vi "灰度图像平滑去毛刺处理.vi"(9 "滤波方法选择":enum16{"中值滤波", "平滑滤波"}(ring), 11 "Image":T1) -> (3 "Image Out":T1)   [LabVIEW 2018]
uses:
  <vilib>/vision/Image Controls.llb/IMAQ Image.ctl
  <vilib>/vision/NI_Vision_Development_Module.lvlib
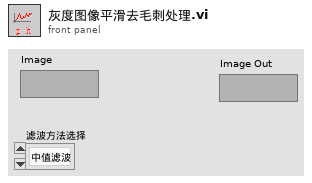
[diagram p1: front panel]
types:
  T1 = typedef "IMAQ Image.ctl" = refnum<image>
  T2 = cluster{bool, bool, bool, bool, bool, bool, bool, bool}
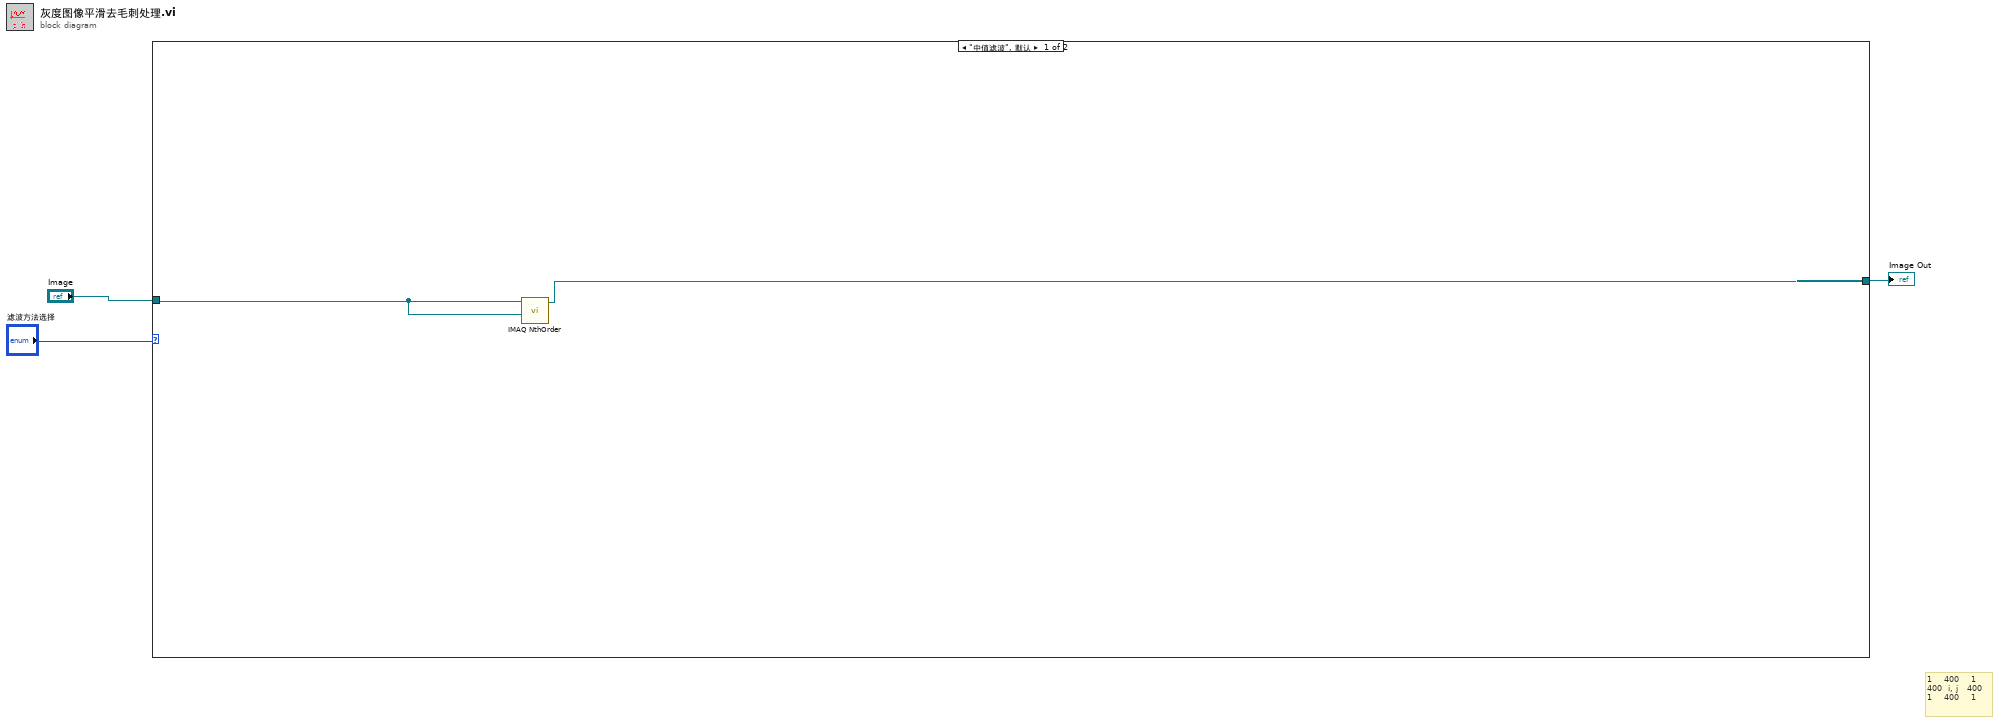
[diagram p0: block diagram]
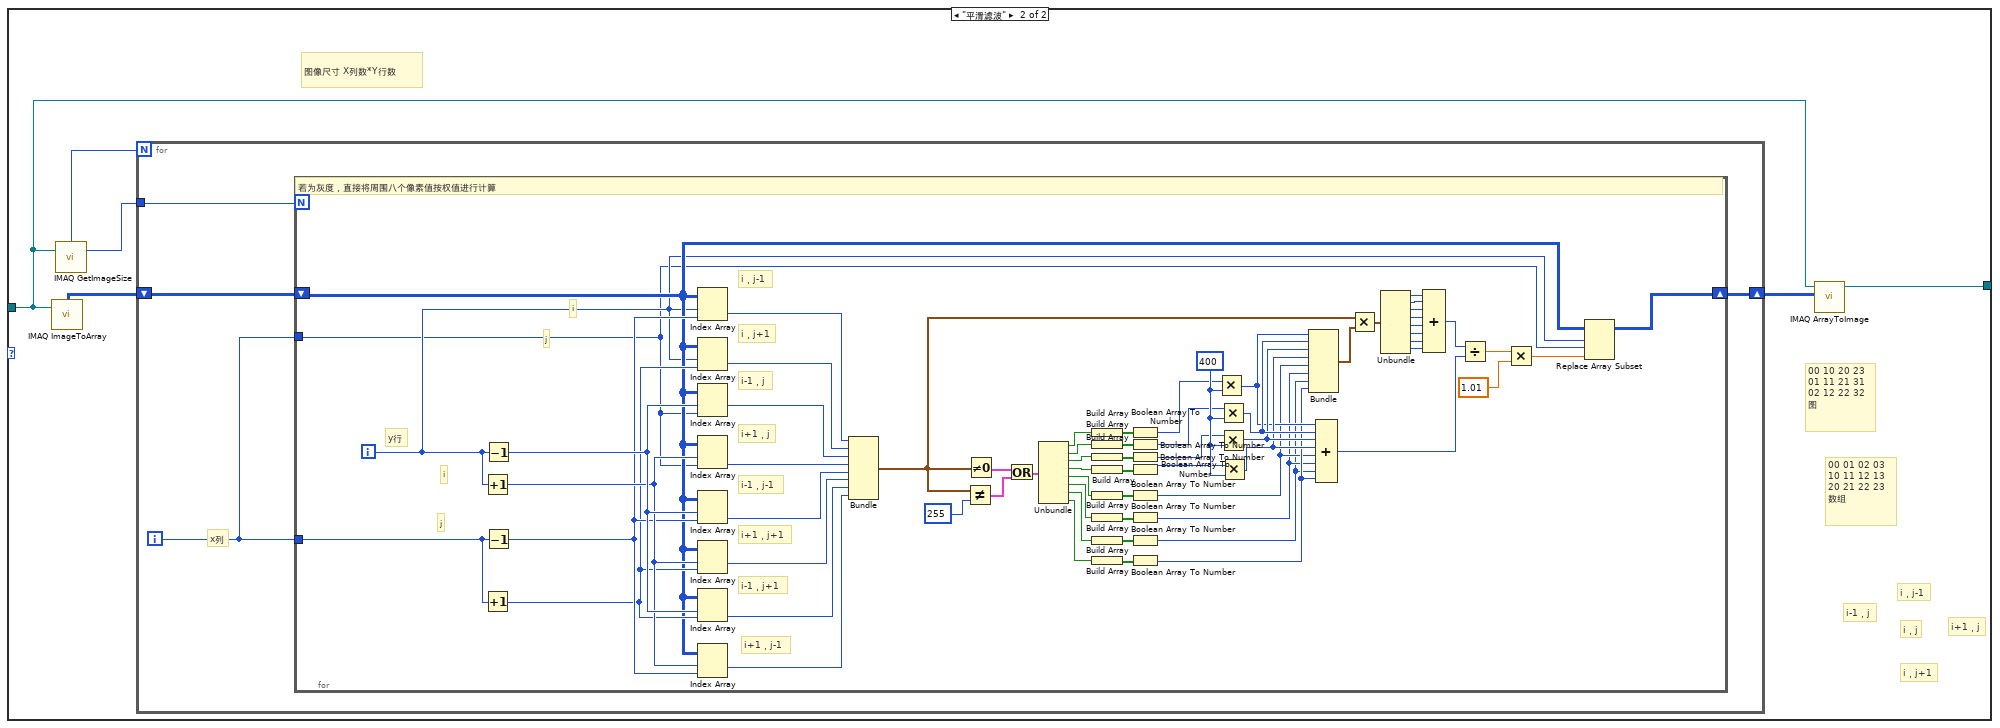
[diagram p2: hidden frame]
diagram:
  # "1    400    1\n400  i, j   400\n1    400    1"
  n1 = case shown="\"中值滤波\", 默认" "滤波方法选择" {
    tunnel: [w4 w11] -> w3
    tunnel: "Image" -> [w5 w8]
    frame "中值滤波", Default {
      n2 = call "IMAQ NthOrder"("Image Src"=w5, "Image Dst"=w5) -> ("Image Dst Out"=w4:T1)  [unwired: 5 in, 1 out]
    }
    frame "平滑滤波" {
      # "i+1，j"
      # "i，j+1"
      # "i，j"
      # "i，j-1"
      # "00 10 20 23\n01 11 21 31\n02 12 22 32\n图"
      # "i-1，j"
      # "00 01 02 03\n10 11 12 13\n20 21 22 23\n数组"
      # "图像尺寸 X列数*Y行数"
      n3 = call "IMAQ ImageToArray"("Image"=w8) -> ("Image Pixels (U8)"=w9:u8[][])  [unwired: 3 in, 4 out]
      n4 = call "IMAQ GetImageSize"("Image"=w8) -> ("Y Resolution"=w7:i32, "X Resolution"=w6:i32)  [unwired: 3 in, 1 out]
      n5 = for {
        N: w6 -> [_]
        shift-right: [w14] -> w10
        shift-left: w9 -> [w15]
        tunnel: w7 -> [w13]
        i -> [w12]
        # "x列"
        n6 = for {
          N: w13 -> [_]
          shift-right: [w79] -> w14
          shift-left: w15 -> [w45]
          tunnel: w12 -> [w78]
          tunnel: w12 -> [w43]
          i -> [w44]
          w75 = u32 400 ("y")
          # "i+1，j-1"
          # "i-1，j+1"
          # "i+1，j+1"
          # "i-1，j-1"
          # "i-1，j"
          # "i+1，j"
          # "i，j+1"
          # "i，j-1"
          # "j"
          # "i"
          # "i"
          # "j"
          # "y行"
          # "若为灰度，直接将周围八个像素值按权值进行计算"
          n7 = Increment(x=w44) -> (x+1=w80:i32)
          n8 = Increment(x=w78) -> (x+1=w76:i32)
          n9 = Decrement(x=w44) -> (x-1=w81:i32)
          n10 = Decrement(x=w78) -> (x-1=w77:i32)
          n11 = Index Array(array=w45, index (row)=w44, index (col)=w77) -> (element=w53:u8)
          n12 = Index Array(array=w45, index (row)=w44, index (col)=w76) -> (element=w52:u8)
          n13 = Index Array(array=w45, index (row)=w81, index (col)=w43) -> (element=w51:u8)
          n14 = Index Array(array=w45, index (row)=w80, index (col)=w43) -> (element=w50:u8)
          n15 = Index Array(array=w45, index (row)=w81, index (col)=w77) -> (element=w49:u8)
          n16 = Index Array(array=w45, index (row)=w80, index (col)=w76) -> (element=w48:u8)
          n17 = Index Array(array=w45, index (row)=w81, index (col)=w76) -> (element=w47:u8)
          n18 = Index Array(array=w45, index (row)=w80, index (col)=w77) -> (element=w46:u8)
          n19 = Bundle(w53, w52, w51, w50, w49, w48, w47, w46) -> (w65:cluster{u8, u8, u8, u8, u8, u8, u8, u8})  [unwired: 1 in]
          n20 = Not Equal?(x=w65, y=u8 255) -> (x != y?=w17:T2)
          n21 = Not Equal To 0?(x=w65) -> (x != 0?=w18:T2)
          n22 = Or(x=w18, y=w17) -> (x .or. y?=w16:T2)
          n23 = Unbundle(w16) -> (w35:bool, w26:bool, w25:bool, w24:bool, w23:bool, w22:bool, w21:bool, w20:bool)
          n24 = Build Array(w35) -> (w34:bool[])
          n25 = Build Array(w26) -> (w33:bool[])
          n26 = Build Array(w25) -> (w32:bool[])
          n27 = Build Array(w24) -> (w31:bool[])
          n28 = Build Array(w23) -> (w27:bool[])
          n29 = Build Array(w22) -> (w28:bool[])
          n30 = Build Array(w21) -> (w29:bool[])
          n31 = Build Array(w20) -> (w30:bool[])
          n32 = Boolean Array To Number(Boolean array=w34) -> (number=w74:u32)
          n33 = Boolean Array To Number(Boolean array=w33) -> (number=w73:u32)
          n34 = Boolean Array To Number(Boolean array=w32) -> (number=w72:u32)
          n35 = Boolean Array To Number(Boolean array=w31) -> (number=w71:u32)
          n36 = Boolean Array To Number(Boolean array=w27) -> (number=w38:u32)
          n37 = Boolean Array To Number(Boolean array=w28) -> (number=w37:u32)
          n38 = Boolean Array To Number(Boolean array=w29) -> (number=w36:u32)
          n39 = Boolean Array To Number(Boolean array=w30) -> (number=w39:u32)
          n40 = Multiply(x=w74, y=w75) -> (x*y=w67:u32)
          n41 = Multiply(x=w73, y=w75) -> (x*y=w70:u32)
          n42 = Multiply(x=w72, y=w75) -> (x*y=w69:u32)
          n43 = Multiply(x=w71, y=w75) -> (x*y=w68:u32)
          n44 = Bundle(w67, w70, w69, w68, w38, w37, w36, w39) -> (w66:cluster{u32, u32, u32, u32, u32, u32, u32, u32})  [unwired: 1 in]
          n45 = Compound Arithmetic op=ADD(w67, w70, w69, w68, w38, w37, w36, w39) -> (w54:u32)
          n46 = Multiply(x=w65, y=w66) -> (x*y=w64:cluster{u32, u32, u32, u32, u32, u32, u32, u32})
          n47 = Unbundle(w64) -> (w63:u32, w62:u32, w61:u32, w60:u32, w59:u32, w58:u32, w57:u32, w56:u32)
          n48 = Compound Arithmetic op=ADD(w63, w62, w61, w60, w59, w58, w57, w56) -> (w55:u32)
          n49 = Divide(x=w55, y=w54) -> (x/y=w42:dbl)
          n50 = Multiply(x=w42, y=1.01) -> (x*y=w40:dbl)
          n51 = Replace Array Subset(array=w45, new element=w40, index (row)=w44, index (col)=w43) -> (w79:u8[][])
        }
      }
      n52 = call "IMAQ ArrayToImage"("Image Pixels (U8)"=w10, "Image"=w8) -> ("Image Out"=w11:T1)  [unwired: 8 in, 1 out]
    }
  }
  "Image Out" <- w3
